vi "ゲージデータ取り込み_サブ1.vi"(9 "配列指標":i32, 10 "ループ回数数値":i32, 11 "VISA Refnum入力":refnum<visa-resource-name>) -> (0 "エラー出力":errorcluster, 3 "VISA Refnum出力":refnum<visa-resource-name>)   [LabVIEW 2021]
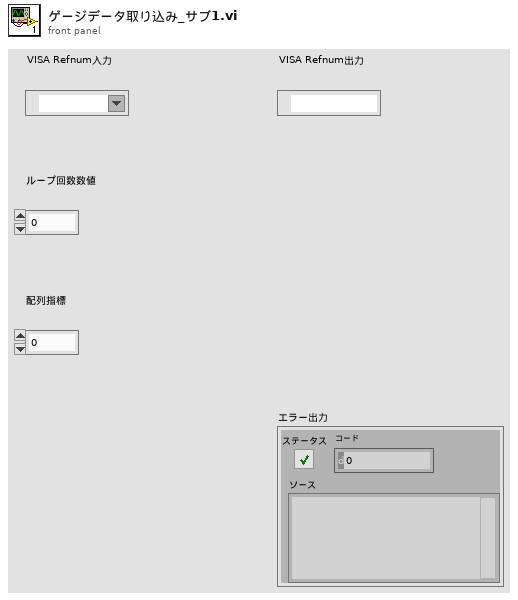
[diagram p1: front panel]
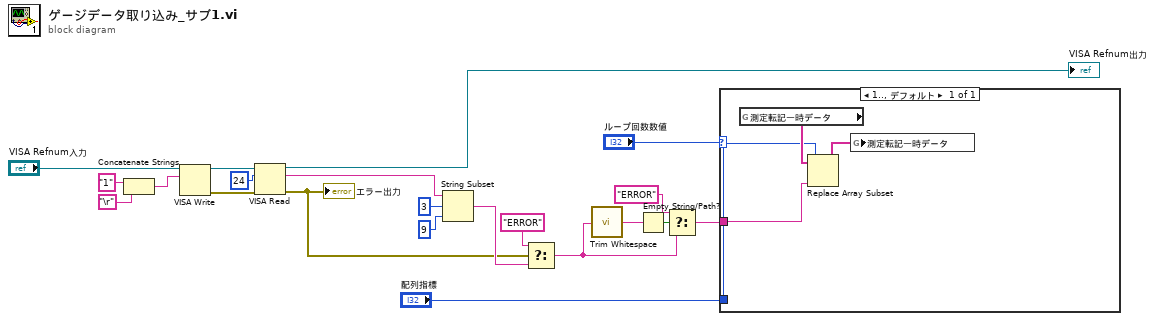
[diagram p0: block diagram]
diagram:
  n1 = Concatenate Strings("1" ("書き込みバッファ"), "\r") -> (w14:string)
  n2 = VISA Write(VISA resource name="VISA Refnum入力", write buffer=w14) -> (VISA resource name out=w15:refnum<visa-resource-name>, error out=w16:errorcluster)  [unwired: 1 in, 1 out]
  n3 = VISA Read(VISA resource name=w15, byte count=u32 24 ("バイトカウント"), error in (no error)=w16) -> (VISA resource name out=→"VISA Refnum出力":refnum<visa-resource-name>, read buffer=w7:string, error out=w2:errorcluster)  [unwired: 1 out]
  "エラー出力" <- w2
  n4 = String Subset(string=w7, offset (0)=3 ("長さ (残り)"), length (rest)=9) -> (substring=w19:string)
  n5 = Select(t="ERROR", s=w2, f=w19) -> (s? t:f=w3:string)
  n6 = call <vilib>:"Trim Whitespace.vi"("string"=w3) -> ("trimmed string"=w4:string)  [unwired: 1 in]
  n7 = Empty String/Path?(string/path=w4) -> (empty?=w8:bool)
  n8 = Select(t="ERROR", s=w8, f=w3) -> (s? t:f=w9:string)
  n9 = case shown="1.., デフォルト" "ループ回数数値" {
    tunnel: w9 -> [w24]
    tunnel: "配列指標" -> [w23]
    frame 1.., Default {
      n10 = global read "測定データ転記.vi" "測定転記一時データ"() -> (w25:string[])
      n11 = Replace Array Subset(array=w25, new element=w24, index=w23) -> (w22:string[])
      n12 = global write "測定データ転記.vi" "測定転記一時データ"(w22) -> ()
    }
  }
